vi "Copy Package.vi"(8 "error in (no error)":errorcluster, 11 "PostBuildSupport in":refnum<class "PostBuildSupport.lvclass">) -> (0 "error out":errorcluster, 3 "PostBuildSupport out":refnum<class "PostBuildSupport.lvclass">)   [LabVIEW 2016, in "PostBuildSupport.lvclass"]
uses:
  PostBuildSupport.lvclass
  PostBuildSupport.lvclass/PostBuildSupport.ctl
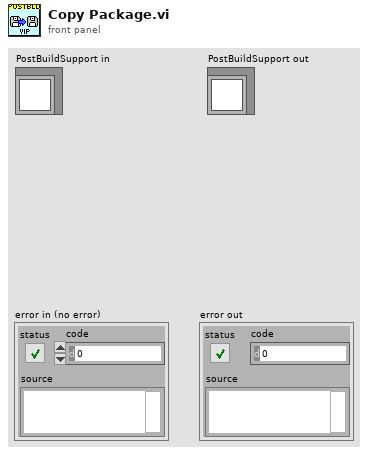
[diagram p1: front panel]
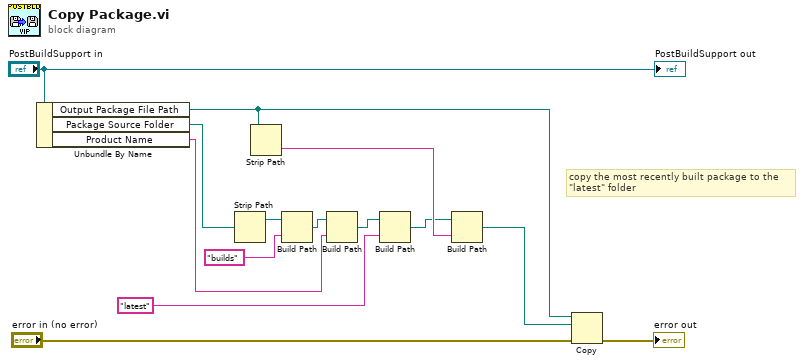
[diagram p0: block diagram]
diagram:
  # "copy the most recently built package to the \n\"latest\" folder"
  n1 = Unbundle By Name("PostBuildSupport in") -> ("Output Package File Path"=w1:path, "Package Source Folder"=w3:path, "Product Name"=w2:string)
  n2 = Strip Path(path=w3) -> (stripped path=w12:path)  [unwired: 1 out]
  n3 = Strip Path(path=w1) -> (name=w11:string)  [unwired: 1 out]
  n4 = Build Path(base path=w12, name or relative path="builds") -> (appended path=w8:path)
  n5 = Build Path(base path=w8, name or relative path=w2) -> (appended path=w7:path)
  n6 = Build Path(base path=w7, name or relative path="latest") -> (appended path=w5:path)
  n7 = Build Path(base path=w5, name or relative path=w11) -> (appended path=w10:path)
  n8 = Copy(8:"error in (no error)", 10:w10, 11:w1) -> (0:→"error out":errorcluster)  [unwired: 2 in, 2 out]
  "PostBuildSupport out" <- "PostBuildSupport in"
